vi "Convert Gap to Goal.vi"(8 "Goal Y":dbl, 11 "Best Known Gap (mm)":cluster{i32, i32}) -> (3 "Goal":cluster{"X":dbl, "Y":dbl})   [LabVIEW 2017]
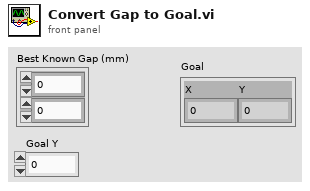
[diagram p1: front panel]
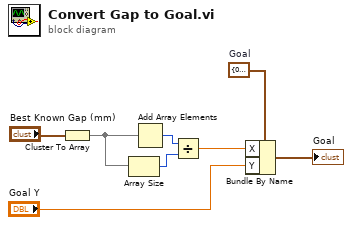
[diagram p0: block diagram]
diagram:
  w7 = cluster{"X":dbl, "Y":dbl} {"X"=0.0, "Y"=0.0}  # Goal
  n1 = Cluster To Array(cluster="Best Known Gap (mm)") -> (array=w2:i32[])
  n2 = Array Size(array=w2) -> (size(s)=w3:i32)
  n3 = Add Array Elements(numeric array=w2) -> (sum=w4:i32)
  n4 = Divide(x=w4, y=w3) -> (x/y=w1:dbl)
  n5 = Bundle By Name(cluster=w7, "X"=w1, "Y"="Goal Y") -> (→"Goal":cluster{"X":dbl, "Y":dbl})
